vi "Check if no Measurement Selected.vi"(8 "error in (no error)":errorcluster, 11 "multicolumnListbox in":refnum<vi>) -> (0 "error out":errorcluster, 1 "warning?":string, 2 "create client disabled?":T1(ring), 3 "multicolumnListbox out":refnum<vi>)   [LabVIEW 2021, in "MeasurementClient Editor.lvlib"]
uses:
  MeasurementClient Editor.lvlib
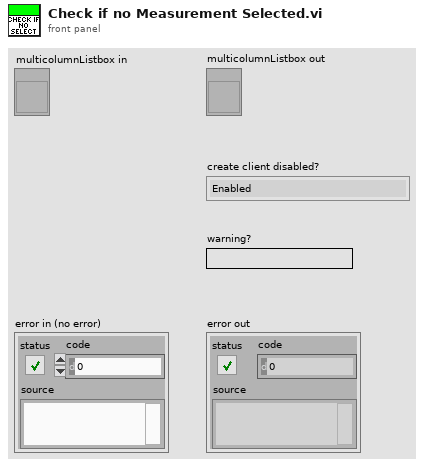
[diagram p1: front panel]
types:
  T1 = enum8{"Enabled", "Disabled", "Disabled and Grayed Out"}
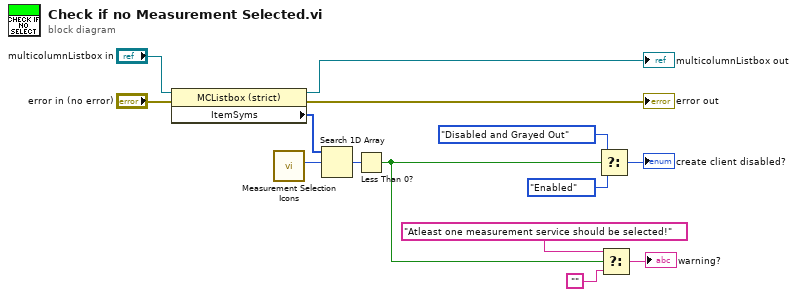
[diagram p0: block diagram]
diagram:
  n1 = property class="MCListbox (strict)"(reference="multicolumnListbox in", error in="error in (no error)") -> (reference out=→"multicolumnListbox out":refnum<vi>, error out=→"error out":errorcluster, "ItemSyms"=w11:i32[])
  n2 = call "Measurement Selection Icons.vi"() -> ("Checked"=w5:i32)  [unwired: 10 in, 1 out]
  n3 = Search 1D Array(1D array=w11, element=w5) -> (index of element=w12:i32)  [unwired: 1 in]
  n4 = Less Than 0?(x=w12) -> (x < 0?=w2:bool)
  n5 = Select(t=T1."Disabled and Grayed Out", s=w2, f=T1."Enabled" ("Disabled")) -> (s? t:f=→"create client disabled?":T1)
  n6 = Select(t="Atleast one measurement service should be selected!", s=w2, f="") -> (s? t:f=→"warning?":string)
